vi "Create FL Channels - XNET CAN.vi"(8 "error in (no error)":errorcluster, 10 "XNET Cluster":refnum<k21>="ManyXnetChannels", 11 "CAN Interface":refnum<k21>="CAN1") -> (0 "error out":errorcluster, 2 "Signal Names":string[](array[string]), 3 "Producer Channels":refnum<class "Producer Channel.lvclass">[](array[class]))   [LabVIEW 2021, in "XNET-CAN-Signal-Logger.lvlib"]
uses:
  XNET-CAN-Signal-Logger.lvlib
  <vilib>/FlexLogger/SDK/PluginSDK.lvlibp/PEFClasses/SDK/Producer Channel/Producer Channel.lvclass
  <vilib>/FlexLogger/SDK/PluginSDK.lvlibp/PEFClasses/SDK/Producer Channel/Create Producer Channel.vi
  <resource>/objmgr/xnet.rc
  <vilib>/FlexLogger/SDK/PluginSDK.lvlibp
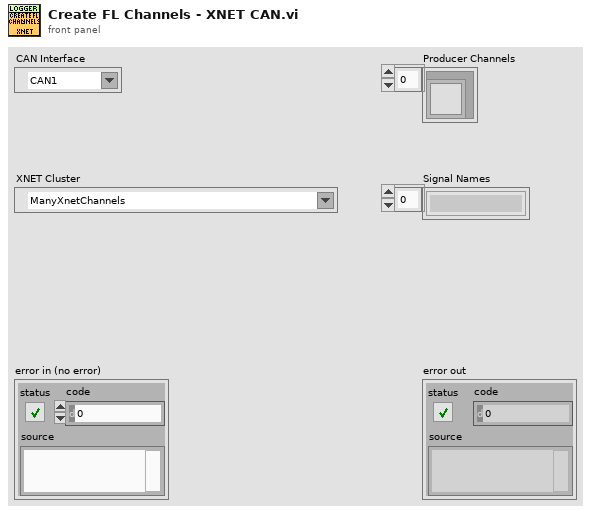
[diagram p1: front panel]
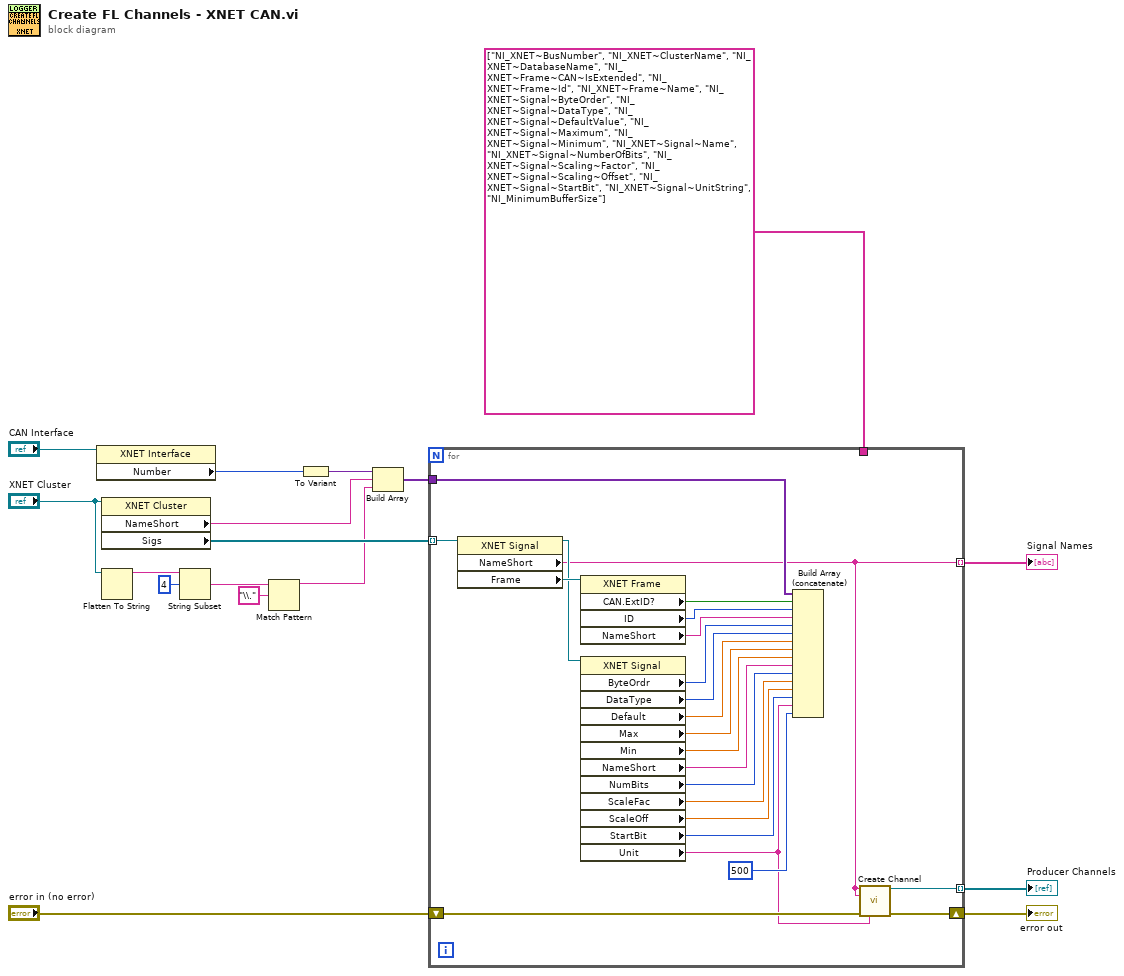
[diagram p0: block diagram]
diagram:
  n1 = property class="XNET Interface"(reference="CAN Interface") -> ("Number"=w11:u32)  [unwired: 1 in, 2 out]
  n2 = property class="XNET Cluster"(reference="XNET Cluster") -> ("NameShort"=w6:string, "Sigs"=w8:refnum<k21>[])  [unwired: 1 in, 2 out]
  n3 = Flatten To String(anything="XNET Cluster") -> (data string=w13:string)  [unwired: 3 in, 2 out]
  n4 = String Subset(string=w13, offset (0)=4) -> (substring=w9:string)  [unwired: 1 in]
  n5 = Match Pattern(string=w9, regular expression="\\.") -> (before substring=w4:string)  [unwired: 1 in, 3 out]
  n6 = To Variant(anything=w11) -> (Variant=w10:variant)
  n7 = Build Array(w10, w6, w4) -> (w7:variant[])
  n8 = for {
    tunnel: w8 -> [w40] mode=indexing
    tunnel: [w21] -> w16 mode=indexing
    tunnel: string[] ["NI_XNET~BusNumber", "NI_XNET~ClusterName", "NI_XNET~DatabaseName", "NI_XNET~Frame~CAN~IsExtended", "NI_XNET~Frame~Id", "NI_XNET~Frame~Name", "NI_XNET~Signal~ByteOrder", "NI_XNET~Signal~DataType", "NI_XNET~Signal~DefaultValue", "NI_XNET~Signal~Maximum", "NI_XNET~Signal~Minimum", "NI_XNET~Signal~Name", "NI_XNET~Signal~NumberOfBits", "NI_XNET~Signal~Scaling~Factor", "NI_XNET~Signal~Scaling~Offset", "NI_XNET~Signal~StartBit", "NI_XNET~Signal~UnitString", "NI_MinimumBufferSize"] ("property names") -> [_]
    tunnel: w7 -> [w37]
    shift-right: [w19] -> w2
    shift-left: "error in (no error)" -> [w22]
    tunnel: [w18] -> w1 mode=indexing
    n9 = property class="XNET Signal"(reference=w40) -> (reference out=w38:refnum<k21>, "NameShort"=w21:string, "Frame"=w39:refnum<k21>)  [unwired: 1 in, 1 out]
    n10 = property class="XNET Frame"(reference=w39) -> ("CAN.ExtID?"=w36:bool, "ID"=w35:u32, "NameShort"=w34:string)  [unwired: 1 in, 2 out]
    n11 = property class="XNET Signal"(reference=w38) -> ("ByteOrdr"=w33:u32, "DataType"=w32:u32, "Default"=w31:dbl, "Max"=w30:dbl, "Min"=w29:dbl, "NameShort"=w28:string, "NumBits"=w27:u32, "ScaleFac"=w26:dbl, "ScaleOff"=w25:dbl, "StartBit"=w24:u32, "Unit"=w20:string)  [unwired: 1 in, 2 out]
    n12 = Build Array (concatenate)(w37, w36, w35, w34, w33, w32, w31, w30, w29, w28, w27, w26, w25, w24, w20, u32 500 ("Start Bit")) -> ()  [unwired: 1 out]
    n13 = call-poly <vilib>:"Create Channel.vi"("Unique Channel Identifier"=w21, "Default Channel Name"=w21, "error in (no error)"=w22, "Unit"=w20) -> ("Producer Channel"=w18:refnum<class "Producer Channel.lvclass">, "error out"=w19:errorcluster)  [unwired: 10 in]
  }
  "error out" <- w2
  "Signal Names" <- w16
  "Producer Channels" <- w1
